vi "Reveal.vi"(8 "error in (no error)":errorcluster, 10 "Result":u32[](array[colorbox]), 11 "View in":refnum<class "View.lvclass">) -> (0 "error out":errorcluster, 3 "View out":refnum<class "View.lvclass">)   [LabVIEW 2024, in "GUI.lvlib" / "View.lvclass"]
uses:
  View.lvclass
  View.lvclass/View.ctl
  TypeDefs/White.ctl
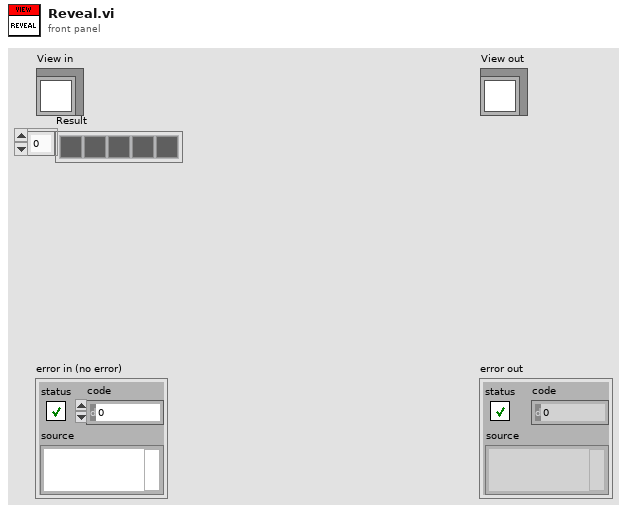
[diagram p1: front panel]
types:
  T1 = typedef "White.ctl" = u32
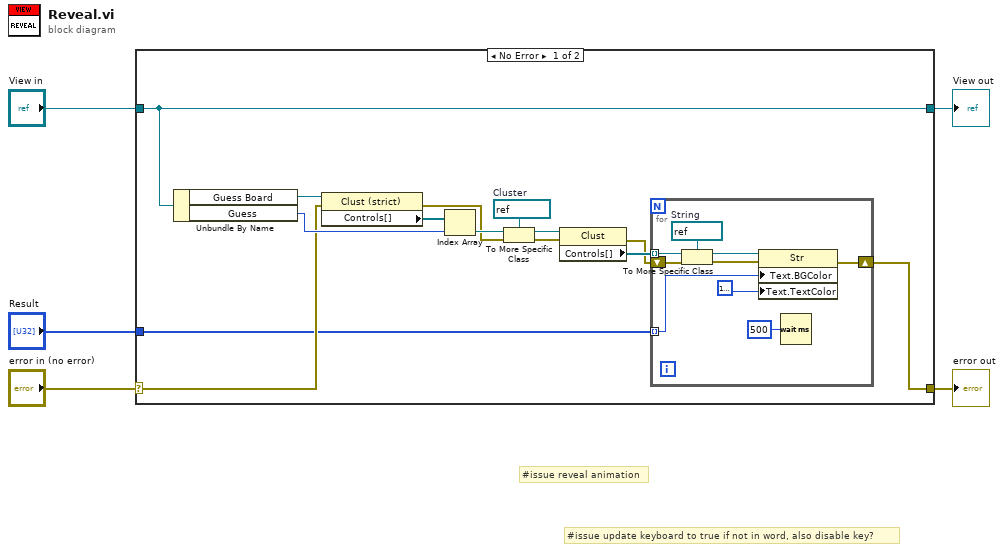
[diagram p0: block diagram]
diagram:
  # "#issue update keyboard to true if not in word, also disable key?"
  # "#issue reveal animation"
  n1 = case shown="No Error" "error in (no error)" {
    selector: "error in (no error)" -> [w9 w30]
    tunnel: [w7 w30] -> w2
    tunnel: [w19 w29] -> w4
    tunnel: "View in" -> [w19 w29]
    tunnel: "Result" -> [w6 _]
    frame No Error {
      w14 = refnum<vi> refnum  # Cluster
      n2 = Unbundle By Name(w19) -> ("Guess Board"=w18:refnum<vi>, "Guess"=w16:i32)
      n3 = property class="Clust (strict)"(reference=w18, error in=w9) -> (error out=w11:errorcluster, "Controls[]"=w17:refnum<vi>[])  [unwired: 1 out]
      n4 = Index Array(array=w17, index=w16) -> (element=w15:refnum<vi>)
      n5 = To More Specific Class(target class=w14, reference=w15, error in=w11) -> (specific class reference=w13:refnum<vi>, error out=w10:errorcluster)
      n6 = property class="Clust"(reference=w13, error in=w10) -> (error out=w8:errorcluster, "Controls[]"=w12:refnum<vi>[])  [unwired: 1 out]
      n7 = for {
        tunnel: w12 -> [w27] mode=indexing
        shift-right: [w25] -> w7
        shift-left: w8 -> [w24]
        tunnel: w6 -> [w22] mode=indexing
        w28 = refnum<vi> refnum  # String
        n8 = To More Specific Class(target class=w28, reference=w27, error in=w24) -> (specific class reference=w26:refnum<vi>, error out=w23:errorcluster)
        n9 = property class="Str"(reference=w26, error in=w23, "Text.BGColor"=w22, "Text.TextColor"=T1 16777225 ("White")) -> (error out=w25:errorcluster)  [unwired: 1 out]
        n10 = Wait (ms)(milliseconds to wait=u32 500) -> ()  [unwired: 1 out]
      }
    }
    frame Error {
    }
  }
  "error out" <- w2
  "View out" <- w4
